vi "PhotonPoseEstimator_Execute_OLD.vi"(7 "Configuration":T12={"Primary Strategy"=enum."LOWEST_AMBIGUITY", "Camera"="", "Initial Pose"={"Translation3d"={"X"=0.0, "Y"=0.0, "Z"=0.0}, "Rotation3d"={"Q_quaternion"={"R"=1.0, "V"=[0.0, 0.0, 0.0]}}}, "HighestAmbiguity"=0.0, "RobotToCamera"={"TRANSLATION3D"={"X"=0.0, "Y"=0.0, "Z"=0.0}, "ROTATION3D"={"Q_quaternion"={"R"=1.0, "V"=[0.0, 0.0, 0.0]}}, "XF"=FALSE}, "FallBack Strategy"=enum."LOWEST_AMBIGUITY", "BaseNTName"="/photonvision"} {"RobotToCamera"."TRANSLATION3D"."Z" format="%14.3f"; "RobotToCamera"."TRANSLATION3D"."Y" format="%14.3f"; "RobotToCamera"."TRANSLATION3D"."X" format="%14.3f"; "Initial Pose"."Translation3d"."Z" format="%14.3f"; "Initial Pose"."Translation3d"."Y" format="%14.3f"; "Initial Pose"."Translation3d"."X" format="%14.3f"}, 8 "AprilTagFieldLayout":T1={"AprilTagMap"={}, "FieldLength"=0.0, "FieldWidth"=0.0, "OriginPosition "=enum."kBlueAllianceWallRightSide,", "OriginPose3d"={"Translation3d"={"X"=0.0, "Y"=0.0, "Z"=0.0}, "Rotation3d"={"Q_quaternion"={"R"=1.0, "V"=[0.0, 0.0, 0.0]}}}} {"OriginPose3d"."Translation3d"."Z" format="%14.3f"; "OriginPose3d"."Translation3d"."Y" format="%14.3f"; "OriginPose3d"."Translation3d"."X" format="%14.3f"}, 9 "ReferencePose":T3={"Translation3d"={"X"=0.0, "Y"=0.0, "Z"=0.0}, "Rotation3d"={"Q_quaternion"={"R"=1.0, "V"=[0.0, 0.0, 0.0]}}} {"Translation3d"."Z" format="%14.3f"; "Translation3d"."Y" format="%14.3f"; "Translation3d"."X" format="%14.3f"}, 10 "PIpeline Has \nNew Results":bool, 11 "PipelineResult":T14={"Targets"=[], "PhotonMultiTargetPNPResult"={"PhotonPNPResult"={"IsPresent"=FALSE, "bestReprojErr"=0.0, "altReprojErr"=0.0, "ambiguity"=0.0, "Best"={"TRANSLATION3D"={"X"=0.0, "Y"=0.0, "Z"=0.0}, "ROTATION3D"={"Q_quaternion"={"R"=1.0, "V"=[0.0, 0.0, 0.0]}}, "XF"=FALSE}, "Alt"={"TRANSLATION3D"={"X"=0.0, "Y"=0.0, "Z"=0.0}, "ROTATION3D"={"Q_quaternion"={"R"=1.0, "V"=[0.0, 0.0, 0.0]}}, "XF"=FALSE}}, "FiducialIDsUsed"=[]}, "PhotonPipelineMetadata"={"CaptureTimestampMicros"=0, "PublishTimestampMicros"=0, "SequenceID"=0, "TimeSinceLastPong"=0}} {"PhotonMultiTargetPNPResult"."PhotonPNPResult"."Alt"."TRANSLATION3D"."Z" format="%14.3f"; "PhotonMultiTargetPNPResult"."PhotonPNPResult"."Alt"."TRANSLATION3D"."Y" format="%14.3f"; "PhotonMultiTargetPNPResult"."PhotonPNPResult"."Alt"."TRANSLATION3D"."X" format="%14.3f"; "PhotonMultiTargetPNPResult"."PhotonPNPResult"."Best"."TRANSLATION3D"."Z" format="%14.3f"; "PhotonMultiTargetPNPResult"."PhotonPNPResult"."Best"."TRANSLATION3D"."Y" format="%14.3f"; "PhotonMultiTargetPNPResult"."PhotonPNPResult"."Best"."TRANSLATION3D"."X" format="%14.3f"; "Targets"."AltCameraToTarget"."TRANSLATION3D"."Z" format="%14.3f"; "Targets"."AltCameraToTarget"."TRANSLATION3D"."Y" format="%14.3f"; "Targets"."AltCameraToTarget"."TRANSLATION3D"."X" format="%14.3f"; "Targets"."BestCameraToTarget"."TRANSLATION3D"."Z" format="%14.3f"; "Targets"."BestCameraToTarget"."TRANSLATION3D"."Y" format="%14.3f"; "Targets"."BestCameraToTarget"."TRANSLATION3D"."X" format="%14.3f"}) -> (0 "TimeStamp_Seconds":dbl, 1 "New Pose Found":bool, 2 "EstimatedPose2d":T8={"TRANSLATION"={"X"=0.0, "Y"=0.0}, "ROTATION"={"VALUE"=0.0, "COS"=1.0, "SIN"=0.0}} {"ROTATION"."SIN" format="%13.4f"; "ROTATION"."COS" format="%13.4f"; "ROTATION"."VALUE" format="%13.4f"; "TRANSLATION"."Y" format="%14.3f"; "TRANSLATION"."X" format="%14.3f"}, 3 "EstimatedPose3d":T3={"Translation3d"={"X"=0.0, "Y"=0.0, "Z"=0.0}, "Rotation3d"={"Q_quaternion"={"R"=1.0, "V"=[0.0, 0.0, 0.0]}}} {"Translation3d"."Z" format="%14.3f"; "Translation3d"."Y" format="%14.3f"; "Translation3d"."X" format="%14.3f"}, 4 "Strategy Used":T11, 5 "PhotonEstimatedRobotPose":T20={"EstimatedPose"={"Translation3d"={"X"=0.0, "Y"=0.0, "Z"=0.0}, "Rotation3d"={"Q_quaternion"={"R"=1.0, "V"=[0.0, 0.0, 0.0]}}}, "TimeStamp_Seconds"=0.0, "targetsUsed"=[], "Strategy"=enum."LOWEST_AMBIGUITY"} {"targetsUsed"."AltCameraToTarget"."TRANSLATION3D"."Z" format="%14.3f"; "targetsUsed"."AltCameraToTarget"."TRANSLATION3D"."Y" format="%14.3f"; "targetsUsed"."AltCameraToTarget"."TRANSLATION3D"."X" format="%14.3f"; "targetsUsed"."BestCameraToTarget"."TRANSLATION3D"."Z" format="%14.3f"; "targetsUsed"."BestCameraToTarget"."TRANSLATION3D"."Y" format="%14.3f"; "targetsUsed"."BestCameraToTarget"."TRANSLATION3D"."X" format="%14.3f"; "EstimatedPose"."Translation3d"."Z" format="%14.3f"; "EstimatedPose"."Translation3d"."Y" format="%14.3f"; "EstimatedPose"."Translation3d"."X" format="%14.3f"}, 6 "out PhotonPoseEstimator":T21={"LastPose"={"Translation3d"={"X"=0.0, "Y"=0.0, "Z"=0.0}, "Rotation3d"={"Q_quaternion"={"R"=1.0, "V"=[0.0, 0.0, 0.0]}}}, "ReferencePose"={"Translation3d"={"X"=0.0, "Y"=0.0, "Z"=0.0}, "Rotation3d"={"Q_quaternion"={"R"=1.0, "V"=[0.0, 0.0, 0.0]}}}, "FieldTags"={"AprilTagMap"={}, "FieldLength"=0.0, "FieldWidth"=0.0, "OriginPosition "=enum."kBlueAllianceWallRightSide,", "OriginPose3d"={"Translation3d"={"X"=0.0, "Y"=0.0, "Z"=0.0}, "Rotation3d"={"Q_quaternion"={"R"=1.0, "V"=[0.0, 0.0, 0.0]}}}}, "PrimaryStratety"=enum."LOWEST_AMBIGUITY", "Camera"="", "RobotToCamera"={"TRANSLATION3D"={"X"=0.0, "Y"=0.0, "Z"=0.0}, "ROTATION3D"={"Q_quaternion"={"R"=1.0, "V"=[0.0, 0.0, 0.0]}}, "XF"=FALSE}, "ReportedErrors"=[], "HighestAmbiguity"=10.0, "MultiTagFallbackStrategy"=enum."LOWEST_AMBIGUITY", "PoseCacheTimeoutSec"=-1.0, "PhotonTargetModel"={"Vertices"=[], "IsPlaner"=FALSE, "IsSpherical"=FALSE}, "BaseNTName"="/photonvision"} {"PhotonTargetModel"."Vertices"."Z" format="%14.3f"; "PhotonTargetModel"."Vertices"."Y" format="%14.3f"; "PhotonTargetModel"."Vertices"."X" format="%14.3f"; "RobotToCamera"."TRANSLATION3D"."Z" format="%14.3f"; "RobotToCamera"."TRANSLATION3D"."Y" format="%14.3f"; "RobotToCamera"."TRANSLATION3D"."X" format="%14.3f"; "FieldTags"."OriginPose3d"."Translation3d"."Z" format="%14.3f"; "FieldTags"."OriginPose3d"."Translation3d"."Y" format="%14.3f"; "FieldTags"."OriginPose3d"."Translation3d"."X" format="%14.3f"; "ReferencePose"."Translation3d"."Z" format="%14.3f"; "ReferencePose"."Translation3d"."Y" format="%14.3f"; "ReferencePose"."Translation3d"."X" format="%14.3f"; "LastPose"."Translation3d"."Z" format="%14.3f"; "LastPose"."Translation3d"."Y" format="%14.3f"; "LastPose"."Translation3d"."X" format="%14.3f"})   [LabVIEW 2019, in "PhotonVisionLib.lvlib"]
doc: "Provided data from polling a camera, update the estimated position of the robot. Returns empty if there are no cameras set or no targets were found from the cameras. \n\nInputs:\n -- PhotonPoseEstimator -- data cluster -- Data guiding how the position determination is done.\n -- PipelineResults -- data cluster -- Data provided from PhotonCamera_GetLatestResults.\n -- HasResults -- boolean - TRUE if targets have been identified in the Pipeline results. This can be provided by PhotonCamera_GetLatestResults.\n\nOutputs:\n - EstimatedPose3d - Pose3d - Estimated 3d position. Only value if NewPoseFound = TRUE\n - EstimatedPose2d - Pose2d - Estimated 2d position. Only value if NewPoseFound = TRUE\n - NewPoseFound -- boolean -- A new position has been determined.\n - TimeStampe - double - Target timestamp (seconds)\n - StrategyUsed -- enum -- The strategy used to determine the pose.\n - PhotonEstimatedRobotPose -- data cluster -- Complete estimated robot position and timestamp data cluster\n -- PhotonPoseEstimator -- data cluster -- Updated data cluster."
uses:
  PhotonVisionLib.lvlib
  <vilib>/Rock Robotics/WPI/ThirdParty/JAS_Junk/TrajLib/Trajectory_Library.lvlib
  <vilib>/Rock Robotics/WPI/ThirdParty/JAS_Junk/TrajLib/TypeDef/TRANSLATION3D.ctl
  <vilib>/Rock Robotics/WPI/ThirdParty/JAS_Junk/TrajLib/TypeDef/QUATERNION.ctl
  <vilib>/Rock Robotics/WPI/ThirdParty/JAS_Junk/TrajLib/TypeDef/ROTATION3D.ctl
  <vilib>/Rock Robotics/WPI/ThirdParty/JAS_Junk/TrajLib/TypeDef/TRANSFORM3D.ctl
  <vilib>/Rock Robotics/WPI/ThirdParty/JAS_Junk/TrajLib/TypeDef/POSE3D.ctl
  <vilib>/Rock Robotics/WPI/ThirdParty/JAS_Junk/TrajLib/TypeDef/AprilTag.ctl
  <vilib>/Rock Robotics/WPI/ThirdParty/JAS_Junk/TrajLib/Enum/AprilTagFieldLayoutOrignPosition_ENUM.ctl
  <vilib>/Rock Robotics/WPI/ThirdParty/JAS_Junk/TrajLib/TypeDef/AprilTagFieldLayout.ctl
  Enum/PhotonPoseStrategy_ENUM.ctl
  TypeDef/PhotonPoseEstimatorType.ctl
  TypeDef/PhotonEstimatedRobotPoseType.ctl
  TypeDef/TargetCornerType.ctl
  TypeDef/PhotonTrackedTargetType.ctl
  TypeDef/PhotonPipelineResultType.ctl
  TypeDef/PhotonPoseEstimator_Configuration.ctl
  TypeDef/PhotonPNPResultType.ctl
  TypeDef/PhotonMultiTargetPNPResultType.ctl
  TypeDef/PhotonTargetModel.ctl
  <vilib>/Rock Robotics/WPI/ThirdParty/JAS_Junk/TrajLib/TypeDef/TRANSLATION2D.ctl
  <vilib>/Rock Robotics/WPI/ThirdParty/JAS_Junk/TrajLib/TypeDef/ROTATION2D.ctl
  <vilib>/Rock Robotics/WPI/ThirdParty/JAS_Junk/TrajLib/TypeDef/POSE2D.ctl
  TypeDef/PhotonPipelineMetadataType.ctl
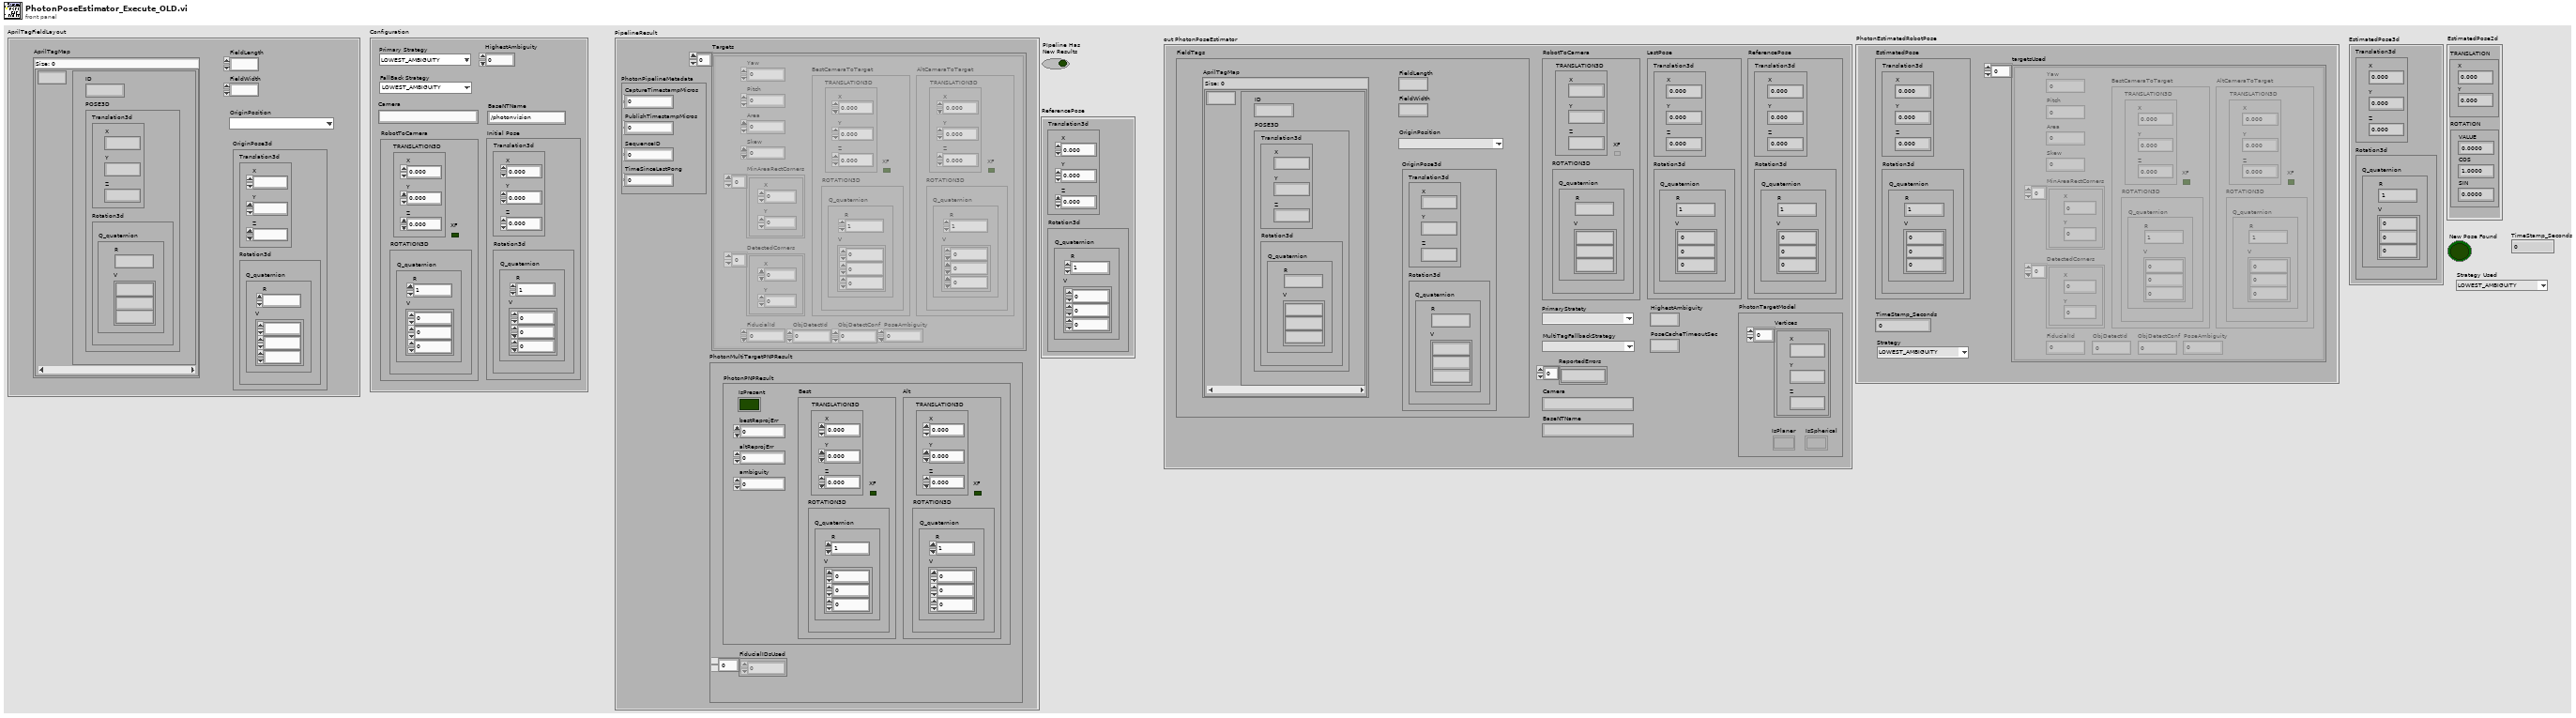
[diagram p1: front panel]
types:
  T1 = typedef "Trajectory_Library.lvlib/AprilTagFieldLayout.ctl" = cluster{"AprilTagMap":map{i32, T2}, "FieldLength":dbl, "FieldWidth":dbl, "OriginPosition ":T7, "OriginPose3d":T3}
  T2 = typedef "Trajectory_Library.lvlib/AprilTag.ctl" = cluster{"ID":i32, "POSE3D":T3}
  T3 = typedef "Trajectory_Library.lvlib/POSE3D.ctl" = cluster{"Translation3d":T4, "Rotation3d":T5}
  T4 = typedef "Trajectory_Library.lvlib/TRANSLATION3D.ctl" = cluster{"X":dbl, "Y":dbl, "Z":dbl}
  T5 = typedef "Trajectory_Library.lvlib/ROTATION3D.ctl" = cluster{"Q_quaternion":T6}
  T6 = typedef "Trajectory_Library.lvlib/QUATERNION.ctl" = cluster{"R":dbl, "V":dbl[]}
  T7 = typedef "Trajectory_Library.lvlib/AprilTagFieldLayoutOrignPosition_ENUM.ctl" = enum16{"kBlueAllianceWallRightSide,", "kRedAllianceWallRightSide,"}
  T8 = typedef "Trajectory_Library.lvlib/POSE2D.ctl" = cluster{"TRANSLATION":T9, "ROTATION":T10}
  T9 = typedef "Trajectory_Library.lvlib/TRANSLATION2D.ctl" = cluster{"X":dbl, "Y":dbl}
  T10 = typedef "Trajectory_Library.lvlib/ROTATION2D.ctl" = cluster{"VALUE":dbl, "COS":dbl, "SIN":dbl}
  T11 = typedef "PhotonVisionLib.lvlib/PhotonPoseStrategy_ENUM.ctl" = enum16{"LOWEST_AMBIGUITY", "CLOSEST_TO_CAMERA_HEIGHT", "CLOSEST_TO_REFERENCE_POSE", "CLOSEST_TO_LAST_POSE", "AVERAGE_BEST_TARGETS", "MULTI_TAG_PNP_ON_COPROCESSOR", "MULTI_TAG_PNP_ON_RIO"}
  T12 = typedef "PhotonVisionLib.lvlib/PhotonPoseEstimator_Configuration.ctl" = cluster{"Primary Strategy":T11, "Camera":string, "Initial Pose":T3, "HighestAmbiguity":dbl, "RobotToCamera":T13, "FallBack Strategy":T11, "BaseNTName":string}
  T13 = typedef "Trajectory_Library.lvlib/TRANSFORM3D.ctl" = cluster{"TRANSLATION3D":T4, "ROTATION3D":T5, "XF":bool}
  T14 = typedef "PhotonVisionLib.lvlib/PhotonPipelineResultType.ctl" = cluster{"Targets":T15[], "PhotonMultiTargetPNPResult":T17, "PhotonPipelineMetadata":T19}
  T15 = typedef "PhotonVisionLib.lvlib/PhotonTrackedTargetType.ctl" = cluster{"Yaw":dbl, "Pitch":dbl, "Area":dbl, "Skew":dbl, "MinAreaRectCorners":T16[], "BestCameraToTarget":T13, "FiducialId":i32, "AltCameraToTarget":T13, "PoseAmbiguity":dbl, "DetectedCorners":T16[], "ObjDetectId":i32, "ObjDetectConf":sgl}
  T16 = typedef "PhotonVisionLib.lvlib/TargetCornerType.ctl" = cluster{"X":dbl, "Y":dbl}
  T17 = typedef "PhotonVisionLib.lvlib/PhotonMultiTargetPNPResultType.ctl" = cluster{"PhotonPNPResult":T18, "FiducialIDsUsed":i16[]}
  T18 = typedef "PhotonVisionLib.lvlib/PhotonPNPResultType.ctl" = cluster{"IsPresent":bool, "bestReprojErr":dbl, "altReprojErr":dbl, "ambiguity":dbl, "Best":T13, "Alt":T13}
  T19 = typedef "PhotonVisionLib.lvlib/PhotonPipelineMetadataType.ctl" = cluster{"CaptureTimestampMicros":i64, "PublishTimestampMicros":i64, "SequenceID":i64, "TimeSinceLastPong":i64}
  T20 = typedef "PhotonVisionLib.lvlib/PhotonEstimatedRobotPoseType.ctl" = cluster{"EstimatedPose":T3, "TimeStamp_Seconds":dbl, "targetsUsed":T15[], "Strategy":T11}
  T21 = typedef "PhotonVisionLib.lvlib/PhotonPoseEstimatorType.ctl" = cluster{"LastPose":T3, "ReferencePose":T3, "FieldTags":T1, "PrimaryStratety":T11, "Camera":string, "RobotToCamera":T13, "ReportedErrors":dbl[], "HighestAmbiguity":dbl, "MultiTagFallbackStrategy":T11, "PoseCacheTimeoutSec":dbl, "PhotonTargetModel":T22, "BaseNTName":string}
  T22 = typedef "PhotonVisionLib.lvlib/PhotonTargetModel.ctl" = cluster{"Vertices":T4[], "IsPlaner":bool, "IsSpherical":bool}
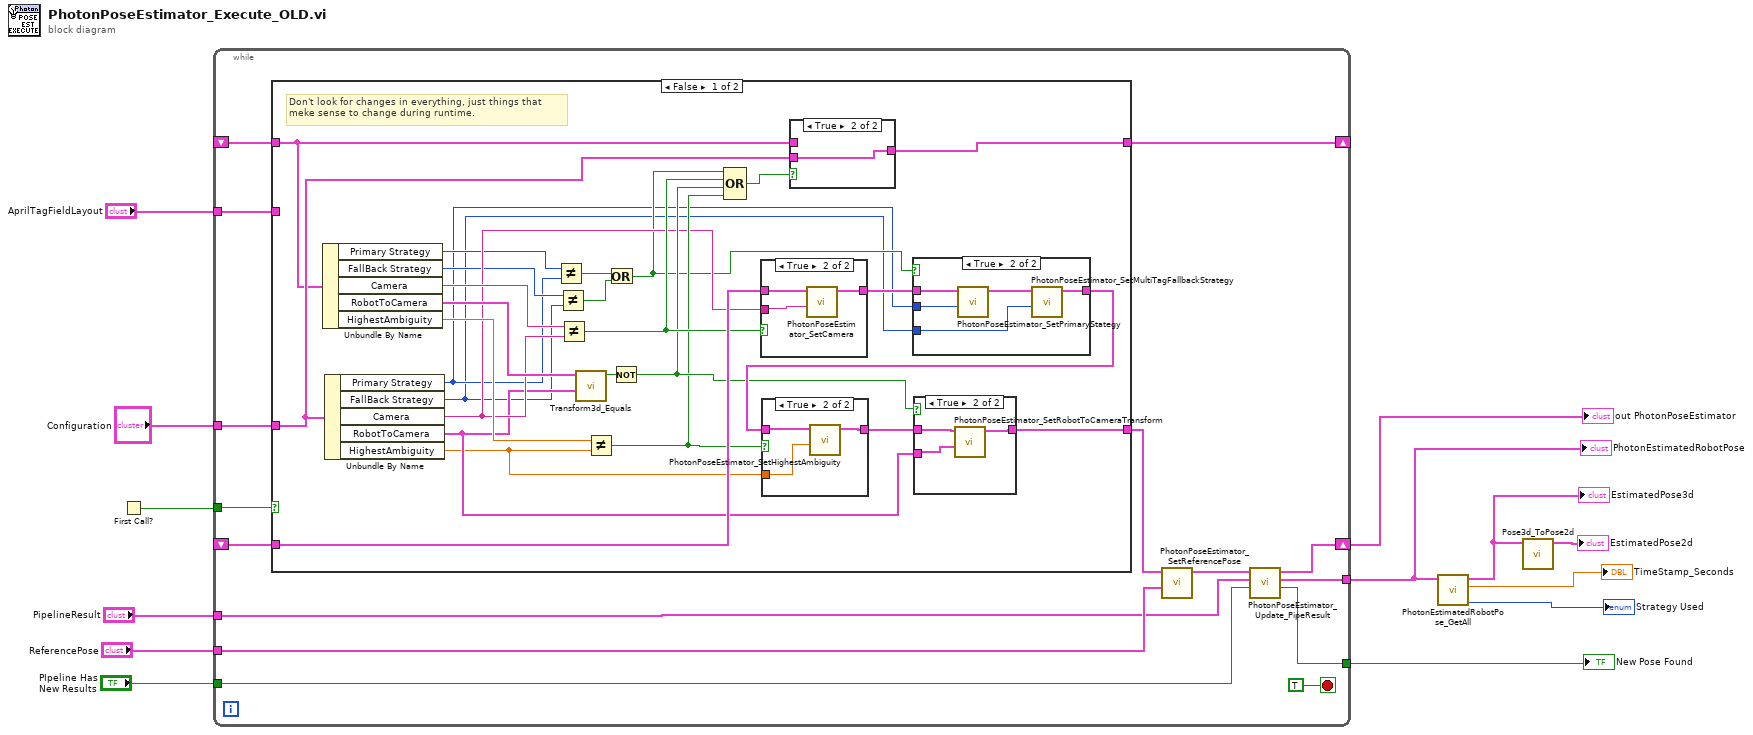
[diagram p0: block diagram]
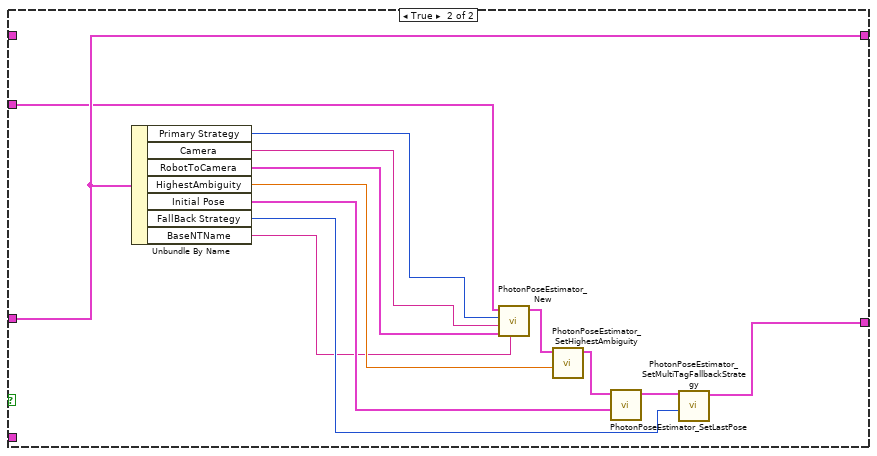
[diagram p7: hidden frame]
diagram:
  n1 = First Call?() -> (First Call?: T/F=w13:bool)
  n2 = while {
    tunnel: w13 -> [w15]
    tunnel: "PipelineResult" -> [w24]
    shift-right: [w22] -> w9
    shift-left: _ -> [w27]
    tunnel: "ReferencePose" -> [w26]
    tunnel: "PIpeline Has \nNew Results" -> [w23]
    tunnel: [w21] -> w6
    tunnel: [w19] -> w8
    tunnel: "Configuration" -> [w17]
    shift-right: [w18] -> _
    shift-left: _ -> [w16]
    tunnel: "AprilTagFieldLayout" -> [w14]
    stop <- TRUE stop-if-true
    n3 = case shown="False" w15 {
      tunnel: [w36 w78] -> w20
      tunnel: w27 -> [w48 _]
      tunnel: w17 -> [w51 w80]
      tunnel: [w49 w80] -> w18
      tunnel: w16 -> [w50 _]
      tunnel: w14 -> [_ w75]
      frame False {
        # "Don't look for changes in everything, just things that\nmeke sense to change during runtime."
        n4 = Unbundle By Name(w50) -> ("Primary Strategy"=w32:T11, "FallBack Strategy"=w31:T11, "Camera"=w45:string, "RobotToCamera"=w41:T13, "HighestAmbiguity"=w54:dbl)
        n5 = Unbundle By Name(w51) -> ("Primary Strategy"=w30:T11, "FallBack Strategy"=w29:T11, "Camera"=w39:string, "RobotToCamera"=w38:T13, "HighestAmbiguity"=w37:dbl)
        n6 = Not Equal?(x=w32, y=w30) -> (x != y?=w34:bool)
        n7 = Not Equal?(x=w31, y=w29) -> (x != y?=w33:bool)
        n8 = Not Equal?(x=w45, y=w39) -> (x != y?=w46:bool)
        n9 = call <vilib>:"Transform3d_Equals.vi"("otherTransform3d"=w38, "inTransform3d"=w41) -> ("Equals"=w53:bool)  [unwired: 9 in]
        n10 = Not Equal?(x=w54, y=w37) -> (x != y?=w40:bool)
        n11 = Or(x=w34, y=w33) -> (x .or. y?=w35:bool)
        n12 = Not(x=w53) -> (.not. x?=w42:bool)
        n13 = Compound Arithmetic op=OR(w35, w46, w42, w40) -> (w52:bool)
        n14 = case shown="True" w46 {
          tunnel: w48 -> [w71 w74]
          tunnel: [w71 w73] -> w47
          tunnel: w39 -> [_ w72]
          frame False {
          }
          frame True {
            n15 = call "PhotonPoseEstimator_SetCamera.vi"("Camera"=w72, "PhotonPoseEstimator"=w74) -> ("out PhotonPoseEstimator"=w73:T21)  [unwired: 9 in]
          }
        }
        n16 = case shown="True" w52 {
          tunnel: w51 -> [_ w70]
          tunnel: w50 -> [w69 _]
          tunnel: [w69 w70] -> w49
          frame False {
          }
          frame True {
          }
        }
        n17 = case shown="True" w35 {
          tunnel: w47 -> [w63 w68]
          tunnel: w30 -> [_ w67]
          tunnel: [w63 w65] -> w43
          tunnel: w29 -> [_ w64]
          frame False {
          }
          frame True {
            n18 = call "PhotonPoseEstimator_SetPrimaryStategy.vi"("PrimaryStrategy"=w67, "PhotonPoseEstimator"=w68) -> ("out PhotonPoseEstimator"=w66:T21)  [unwired: 9 in]
            n19 = call "PhotonPoseEstimator_SetMultiTagFallbackStrategy.vi"("FallBack Strategy"=w64, "PhotonPoseEstimator"=w66) -> ("out PhotonPoseEstimator"=w65:T21)  [unwired: 9 in]
          }
        }
        n20 = case shown="True" w40 {
          tunnel: w43 -> [w59 w62]
          tunnel: [w59 w61] -> w44
          tunnel: w37 -> [_ w60]
          frame False {
          }
          frame True {
            n21 = call "PhotonPoseEstimator_SetHighestAmbiguity.vi"("HighestAmbiguity"=w60, "PhotonPoseEstimator"=w62) -> ("out PhotonPoseEstimator"=w61:T21)  [unwired: 9 in]
          }
        }
        n22 = case shown="True" w42 {
          tunnel: w44 -> [w55 w58]
          tunnel: [w55 w57] -> w36
          tunnel: w38 -> [_ w56]
          frame False {
          }
          frame True {
            n23 = call "PhotonPoseEstimator_SetRobotToCameraTransform.vi"("RobotToCameraTransform3d"=w56, "PhotonPoseEstimator"=w58) -> ("out PhotonPoseEstimator"=w57:T21)  [unwired: 9 in]
          }
        }
      }
      frame True {
        n24 = Unbundle By Name(w80) -> ("Primary Strategy"=w85:T11, "Camera"=w84:string, "RobotToCamera"=w83:T13, "HighestAmbiguity"=w82:dbl, "Initial Pose"=w81:T3, "FallBack Strategy"=w77:T11, "BaseNTName"=w76:string)
        n25 = call "PhotonPoseEstimator_New.vi"("BaseNTName"=w76, "RobotToCamera"=w83, "Camera"=w84, "Strategy"=w85, "AprilTagFieldLayout"=w75) -> ("PhotonPoseEstimator"=w87:T21)  [unwired: 6 in]
        n26 = call "PhotonPoseEstimator_SetHighestAmbiguity.vi"("HighestAmbiguity"=w82, "PhotonPoseEstimator"=w87) -> ("out PhotonPoseEstimator"=w86:T21)  [unwired: 9 in]
        n27 = call "PhotonPoseEstimator_SetLastPose.vi"("LastPose"=w81, "PhotonPoseEstimator"=w86) -> ("out PhotonPoseEstimator"=w79:T21)  [unwired: 9 in]
        n28 = call "PhotonPoseEstimator_SetMultiTagFallbackStrategy.vi"("FallBack Strategy"=w77, "PhotonPoseEstimator"=w79) -> ("out PhotonPoseEstimator"=w78:T21)  [unwired: 9 in]
      }
    }
    n29 = call "PhotonPoseEstimator_SetReferencePose.vi"("ReferencePose"=w26, "PhotonPoseEstimator"=w20) -> ("out PhotonPoseEstimator"=w25:T21)  [unwired: 9 in]
    n30 = call "PhotonPoseEstimator_Update_PipeResult.vi"("Has Results"=w23, "PipelineResult"=w24, "PhotonPoseEstimator"=w25) -> ("Pos Found"=w19:bool, "PhotonEstimatedRobotPose"=w21:T20, "out PhotonPoseEstimator"=w22:T21)  [unwired: 6 in]
  }
  "out PhotonPoseEstimator" <- w9
  "PhotonEstimatedRobotPose" <- w6
  "New Pose Found" <- w8
  n31 = call "PhotonEstimatedRobotPose_GetAll.vi"("PhotonEstimatedRobotPose"=w6) -> ("Strategy"=→"Strategy Used":T11, "TimeStamp_Seconds"=→"TimeStamp_Seconds":dbl, "EstimatedPose"=w4:T3)  [unwired: 7 in, 1 out]
  "EstimatedPose3d" <- w4
  n32 = call <vilib>:"Pose3d_ToPose2d.vi"("in Pose3d"=w4) -> ("out Pose2d"=→"EstimatedPose2d":T8)  [unwired: 10 in]
